vi "TP_FGV_UI_Ref.vi"(7 "Enum":T5(ring)=enum."GetValue", 8 "error in (no error)":errorcluster, 10 "Global Variants in":T4) -> (0 "error out":errorcluster, 2 "Global Variants out":T4)   [LabVIEW 2012]
uses:
  controls/TP_Config.ctl
  controls/TP_UI Ref.ctl
  controls/TP_Privileges.ctl
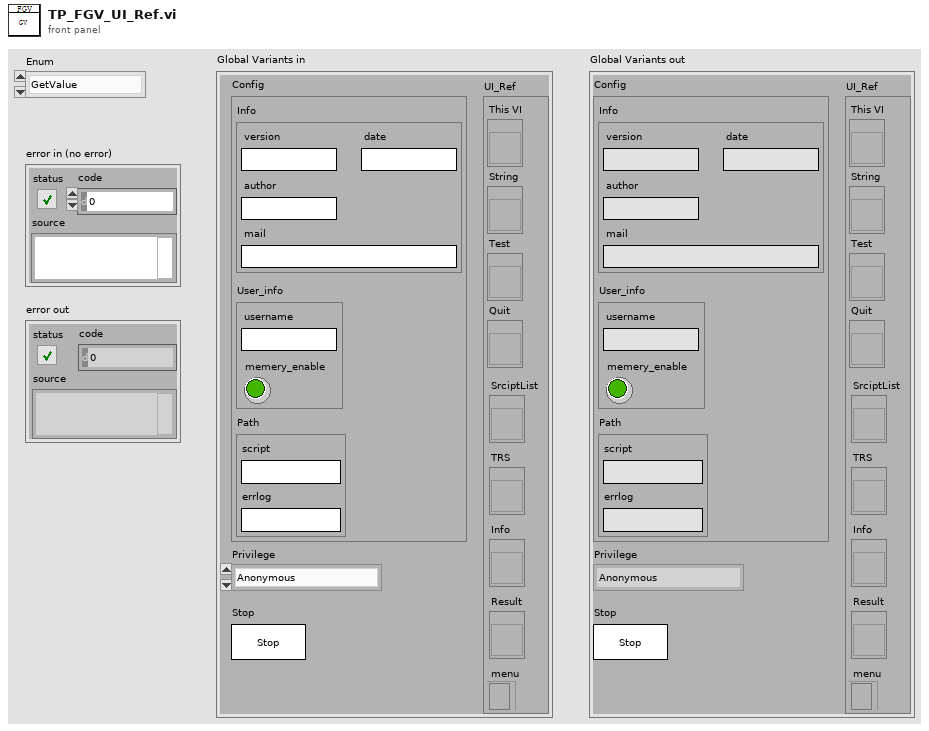
[diagram p1: front panel]
types:
  T1 = typedef "TP_Config.ctl" = cluster{"Info":cluster{"version":string, "date":string, "author":string, "mail":string}, "User_info":cluster{"username":string, "memery_enable":bool}, "Path":cluster{"script":string, "errlog":string}}
  T2 = typedef "TP_UI Ref.ctl" = cluster{"This VI":refnum<vi>, "String":refnum<vi>, "Test":refnum<vi>, "Quit":refnum<vi>, "SrciptList":refnum<vi>, "TRS":refnum<vi>, "Info":refnum<vi>, "Result":refnum<vi>, "menu":refnum<k9>}
  T3 = typedef "TP_Privileges.ctl" = enum16{"Anonymous", "User", "Debugger", "Developer", "Admin"}
  T4 = cluster{"Config":T1, "UI_Ref":T2, "Privilege":T3, "Stop":bool}
  T5 = enum16{"Init", "GetValue", "SetValue", "Destory"}
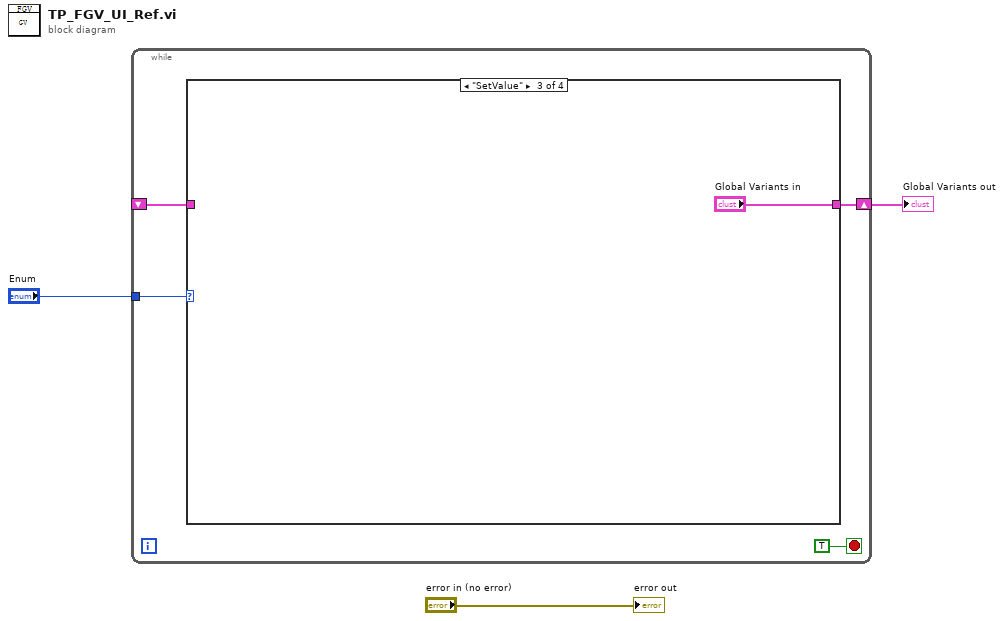
[diagram p0: block diagram]
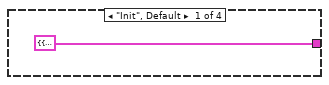
[diagram p2: hidden frame]
diagram:
  n1 = while {
    tunnel: "Enum" -> [w7]
    shift-right: [w5] -> w1
    shift-left: _ -> [w6]
    stop <- TRUE stop-if-true
    n2 = case shown="\"SetValue\"" w7 {
      tunnel: w6 -> [_ w9 _ _]
      tunnel: [T4 {"Config"={"Info"={"version"="", "date"="", "author"="", "mail"=""}, "User_info"={"username"="", "memery_enable"=FALSE}, "Path"={"script"="", "errlog"=""}}, "UI_Ref"={"This VI"=refnum, "String"=refnum, "Test"=refnum, "Quit"=refnum, "SrciptList"=refnum, "TRS"=refnum, "Info"=refnum, "Result"=refnum, "menu"=refnum}, "Privilege"=enum."Anonymous", "Stop"=FALSE} ("Global Variants out") w9 "Global Variants in" _] -> w5
      frame "Init", Default {
      }
      frame "GetValue" {
      }
      frame "SetValue" {
      }
      frame "Destory" {
      }
    }
  }
  "Global Variants out" <- w1
  "error out" <- "error in (no error)"
